vi "Set Configuration.vi"(8 "error in":errorcluster, 10 "transfer settings":T1, 11 "RDMA Transfer Rx Configuration in":refnum<class "RDMA Transfer Rx Configuration.lvclass">=refnum) -> (0 "error out":errorcluster, 3 "RDMA Transfer Rx Configuration out":refnum<class "RDMA Transfer Rx Configuration.lvclass">)   [LabVIEW 2020, in "RDMA.lvlib" / "RDMA Transfer Rx Configuration.lvclass"]
uses:
  RDMA Transfer Rx Configuration.lvclass
  Rx Transfer Settings.ctl
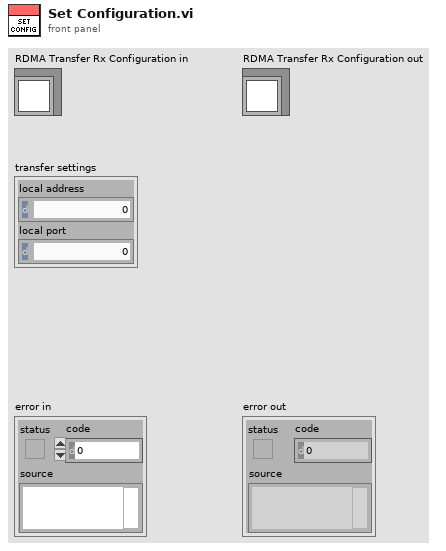
[diagram p1: front panel]
types:
  T1 = typedef "RDMA.lvlib/RDMA Transfer Rx Configuration.lvclass/Rx Transfer Settings.ctl" = cluster{"local address":u32, "local port":u16}
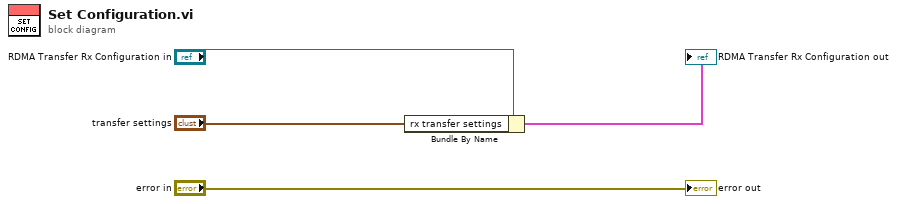
[diagram p0: block diagram]
diagram:
  n1 = Bundle By Name(cluster="RDMA Transfer Rx Configuration in", "rx transfer settings"="transfer settings") -> (→"RDMA Transfer Rx Configuration out":cluster{})
  "error out" <- "error in"
